vi "GetBox.vi"(0 "Path":path=path "/Users/mahevelay/Desktop/EPFL/BA4/prog/projet/198.png", 2 "dark blue frame":T2={"R max"=24, "R min"=0, "G max"=49, "B max"=119, "B min"=100, "G min"=0}, 3 "error in":errorcluster) -> (4 "billard rect":T1, 7 "error out":errorcluster)   [LabVIEW 2021]
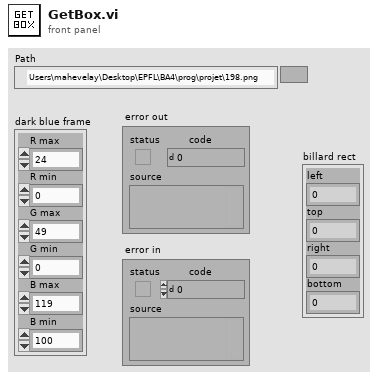
[diagram p1: front panel]
types:
  T1 = cluster{"left":u32, "top":u32, "right":u32, "bottom":u32}
  T2 = cluster{"R max":u8, "R min":u8, "G max":u8, "B max":u8, "B min":u8, "G min":u8}
  T3 = typedef "imagedata.ctl" = cluster{"image type":i32, "image depth":i32, "image":u8[], "mask":u8[], "colors":u32[], "Rectangle":cluster{"left":i16, "top":i16, "right":i16, "bottom":i16}}
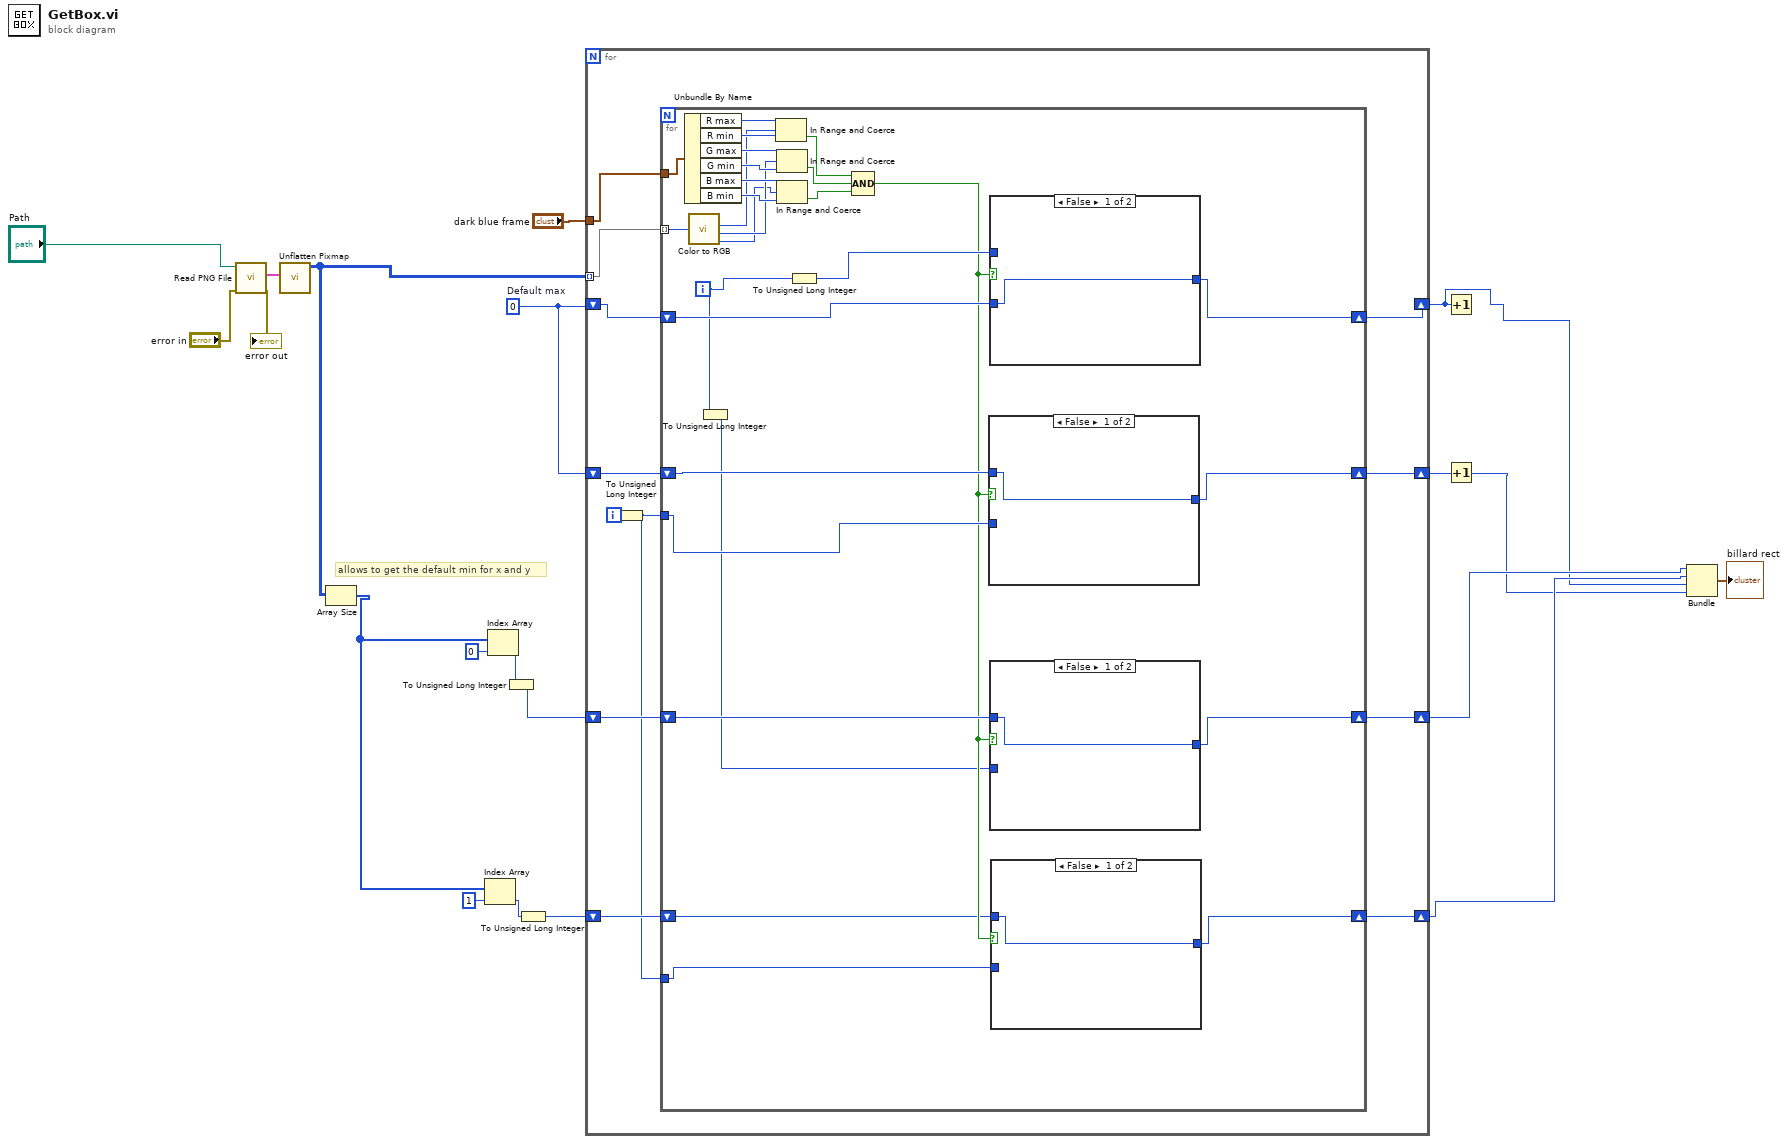
[diagram p0: block diagram]
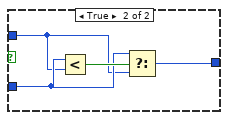
[diagram p2: hidden frame]
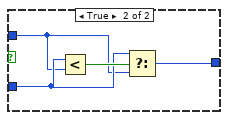
[diagram p3: hidden frame]
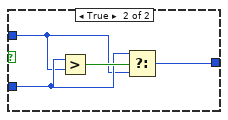
[diagram p4: hidden frame]
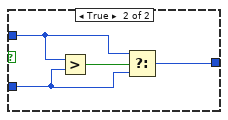
[diagram p5: hidden frame]
diagram:
  w6 = u32 0  # Default max
  # "allows to get the default min for x and y"
  n1 = call <vilib>:"Read PNG File.vi"("error in (no error)"="error in", "path to PNG file"="Path") -> ("error out"=→"error out":errorcluster, "image data"=w19:T3)  [unwired: 7 in, 1 out]
  n2 = call <vilib>:"Unflatten Pixmap.vi"("image data"=w19) -> ("24-bit pixmap"=w9:u32[][])  [unwired: 4 in, 6 out]
  n3 = Array Size(array=w9) -> (size(s)=w14:i32[])
  n4 = Index Array(array=w14, index=1) -> (element=w10:i32)
  n5 = Index Array(array=w14, index=0) -> (element=w11:i32)
  n6 = To Unsigned Long Integer(number=w11) -> (unsigned 32bit integer=w8:u32)
  n7 = To Unsigned Long Integer(number=w10) -> (unsigned 32bit integer=w7:u32)
  n8 = for {
    tunnel: w9 -> [w31] mode=indexing
    tunnel: "dark blue frame" -> [w32]
    shift-right: [w30] -> w16
    shift-left: w6 -> [w29]
    shift-right: [w28] -> w1
    shift-left: w6 -> [w27]
    shift-right: [w25] -> w5
    shift-left: w8 -> [w26]
    shift-right: [w22] -> w4
    shift-left: w7 -> [w23]
    i -> [w24]
    n9 = To Unsigned Long Integer(number=w24) -> (unsigned 32bit integer=w21:u32)
    n10 = for {
      tunnel: w31 -> [w60] mode=indexing
      tunnel: w32 -> [w52]
      shift-right: [w56] -> w28
      shift-left: w27 -> [w41]
      shift-right: [w54] -> w30
      shift-left: w29 -> [w55]
      tunnel: w21 -> [w53]
      shift-right: [w38] -> w25
      shift-left: w26 -> [w40]
      tunnel: w21 -> [w36]
      shift-right: [w34] -> w22
      shift-left: w23 -> [w35]
      i -> [w39]
      n11 = Unbundle By Name(w52) -> ("R max"=w51:u8, "R min"=w50:u8, "G max"=w49:u8, "G min"=w48:u8, "B max"=w47:u8, "B min"=w46:u8)
      n12 = call <vilib>:"Color to RGB.vi"("Color"=w60) -> ("R"=w45:u8, "G"=w44:u8, "B"=w43:u8)  [unwired: 1 out]
      n13 = To Unsigned Long Integer(number=w39) -> (unsigned 32bit integer=w33:u32)
      n14 = In Range and Coerce(upper limit=w51, x=w45, lower limit=w50) -> (In Range?=w59:bool)  [unwired: 1 out]
      n15 = In Range and Coerce(upper limit=w49, x=w44, lower limit=w48) -> (In Range?=w58:bool)  [unwired: 1 out]
      n16 = In Range and Coerce(upper limit=w47, x=w43, lower limit=w46) -> (In Range?=w57:bool)  [unwired: 1 out]
      n17 = To Unsigned Long Integer(number=w39) -> (unsigned 32bit integer=w42:u32)
      n18 = Compound Arithmetic op=AND(w59, w58, w57) -> (w37:bool)
      n19 = case shown="False" w37 {
        tunnel: w55 -> [w71 w72]
        tunnel: w53 -> [_ w73]
        tunnel: [w71 w74] -> w54
        frame False {
        }
        frame True {
          n20 = Greater?(x=w73, y=w72) -> (0:w75:bool)
          n21 = Select(t=w73, s=w75, f=w72) -> (s? t:f=w74:u32)
        }
      }
      n22 = case shown="False" w37 {
        tunnel: w42 -> [_ w79]
        tunnel: w41 -> [w76 w78]
        tunnel: [w76 w77] -> w56
        frame False {
        }
        frame True {
          n23 = Greater?(x=w79, y=w78) -> (0:w80:bool)
          n24 = Select(t=w79, s=w80, f=w78) -> (s? t:f=w77:u32)
        }
      }
      n25 = case shown="False" w37 {
        tunnel: w40 -> [w66 w67]
        tunnel: w33 -> [_ w68]
        tunnel: [w66 w69] -> w38
        frame False {
        }
        frame True {
          n26 = Less?(x=w68, y=w67) -> (x < y?=w70:bool)
          n27 = Select(t=w68, s=w70, f=w67) -> (s? t:f=w69:u32)
        }
      }
      n28 = case shown="False" w37 {
        tunnel: w35 -> [w61 w62]
        tunnel: w36 -> [_ w63]
        tunnel: [w61 w64] -> w34
        frame False {
        }
        frame True {
          n29 = Less?(x=w63, y=w62) -> (x < y?=w65:bool)
          n30 = Select(t=w63, s=w65, f=w62) -> (s? t:f=w64:u32)
        }
      }
    }
  }
  n31 = Increment(x=w1) -> ()  [unwired: 1 out]
  n32 = Increment(x=w16) -> (x+1=w3:u32)
  n33 = Bundle(w5, w4, "Default max"=w1, w3) -> (→"billard rect":cluster{u32, u32, "Default max":u32, u32})  [unwired: 1 in]
